vi "ClassAppData.Delete.vi"(7 "Section":string, 8 "error in (no error)":errorcluster, 10 "Name":string, 11 "Class - App Data in":refnum<class "Class.AppData.lvclass">) -> (0 "error out":errorcluster, 2 "Found":bool, 3 "Class - App Data out":refnum<class "Class.AppData.lvclass">)   [LabVIEW 2024, in "EQMF.lvlib" / "Config Utils.lvlib" / "Class.AppData.lvclass"]
doc: "<B>AppData Class:</B>\nThe AppData class keeps track of a library of data items that are used by an application. These data items have a name (text string) and value that can be any data type. \n\nThis VI is part of the AppData class. This VI will delete the AppData item specified by the Data Name input. \n\nINPUTS:\n<B>Section and Name</B> - The section and name inputs are used to build the name of the item to be set. If only the Name input is populated, then that will be used for the name of the item to set. If both are populated the then the Section and Name will be concatenated with a period separator and that will be used for the name of the item to set.\nEXAMPLE: If Section = \"AA\" and Name = \"BB\" then the name used for the data item will be \"AA.BB\".\n\nOUTPUTS:\n<B>Found</B> - This will be true if the item existed and was removed. \n\n<B>NOTE:</B> If the item specified by Data Name does not exist in the library then this VI will do nothing. No error will be reported."
uses:
  Class.AppData.lvclass
  Class.AppData.lvclass/Class.AppData.ctl
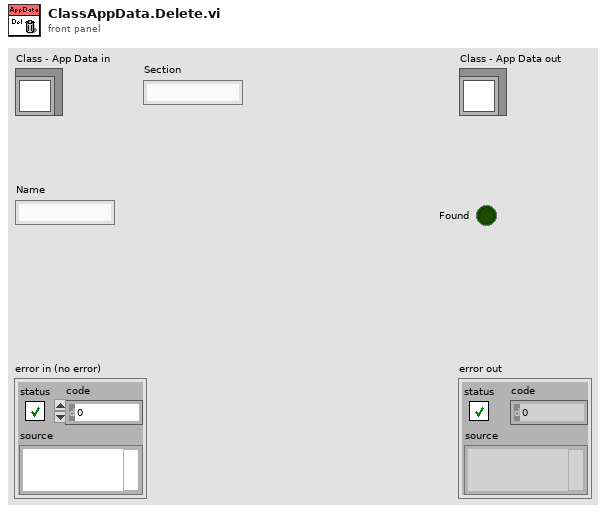
[diagram p1: front panel]
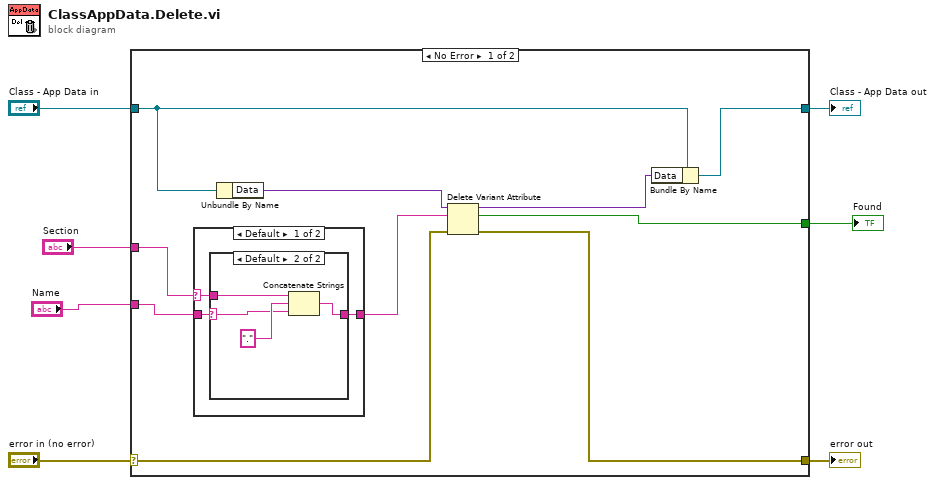
[diagram p0: block diagram]
diagram:
  n1 = case shown="No Error" "error in (no error)" {
    selector: "error in (no error)" -> [w17 w28]
    tunnel: [w15 w28] -> w6
    tunnel: [w11 w27] -> w4
    tunnel: "Class - App Data in" -> [w12 w27]
    tunnel: [w16 _] -> w3
    tunnel: "Section" -> [w9 _]
    tunnel: "Name" -> [w8 _]
    frame No Error {
      n2 = case shown="Default" w9 {
        selector: w9 -> [w20 _]
        tunnel: w8 -> [w18 w26]
        tunnel: [w19 w26] -> w10
        frame Default {
          n3 = case shown="Default" w18 {
            selector: w18 -> [_ w22]
            tunnel: w20 -> [w21 w25]
            tunnel: [w21 w23] -> w19
            frame "" {
            }
            frame Default {
              n4 = Concatenate Strings(w25, ".", w22) -> (w23:string)
            }
          }
        }
        frame "" {
        }
      }
      n5 = Unbundle By Name(w12) -> ("Data"=w14:variant)
      n6 = Delete Variant Attribute(4:w17, 6:w10, 7:w14) -> (0:w15:errorcluster, 2:w16:bool, 3:w13:variant)
      n7 = Bundle By Name(cluster=w12, "Data"=w13) -> (w11:refnum<class "Class.AppData.lvclass">)
    }
    frame Error {
    }
  }
  "error out" <- w6
  "Class - App Data out" <- w4
  "Found" <- w3
